vi "Read Current Probe.vi"(0 "object in":refnum<class "TBS2000Series.lvclass">, 2 "Main Channel":i32(ring)=2 items=["Math", "Channel 1", "Channel 2", "Channel 3", "Channel 4"], 3 "Probe Channel":i32(ring)=3 items=["Math", "Channel 1", "Channel 2", "Channel 3", "Channel 4"], 5 "error in (no error)":errorcluster) -> (14 "object out":refnum<class "TBS2000Series.lvclass">, 15 "Phase Probe":dbl format="%.2p", 16 "Peak-to-Peak Probe":dbl format="%.2p", 19 "error out":errorcluster)   [LabVIEW 2023, in "TBS2000Series.lvclass"]
uses:
  TBS2000Series.lvclass
  TBS2000Series.lvclass/TBS2000Series.ctl
  <instrlib>/Tektronix TBS 2000 Series/Tektronix TBS 2000 Series.lvlib
panel:
  out "Waveform Graph":T1(graph)
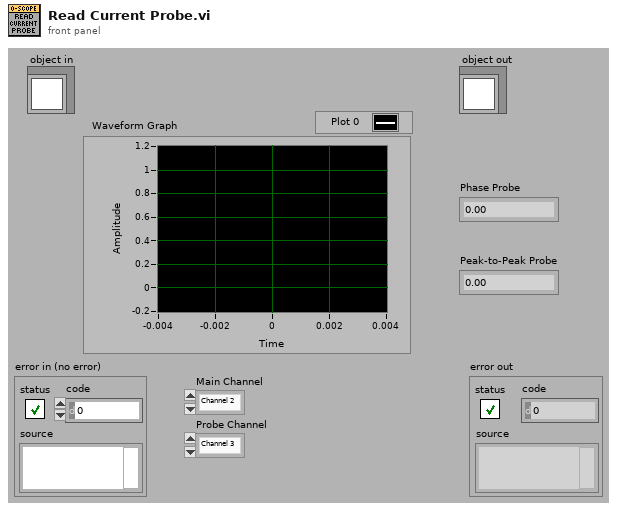
[diagram p1: front panel]
types:
  T1 = cluster{"Initial X":dbl, "X Increment":dbl, "Waveform Array":dbl[]}
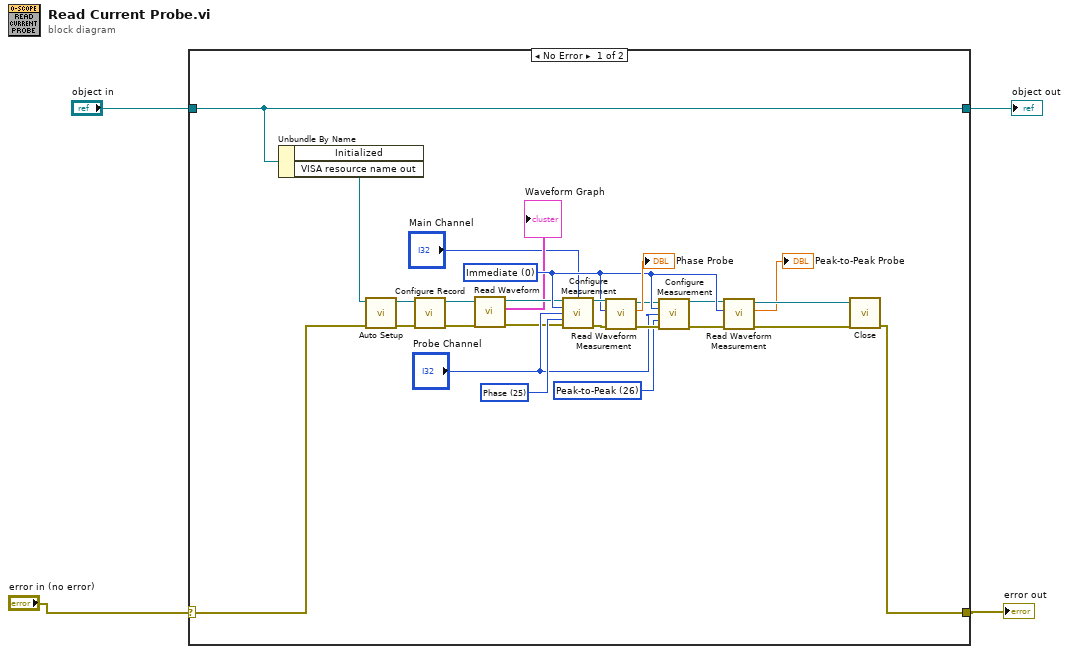
[diagram p0: block diagram]
diagram:
  n1 = case shown="No Error" "error in (no error)" {
    selector: "error in (no error)" -> [w22 w32]
    tunnel: [w21 w32] -> w2
    tunnel: [w23 w31] -> w1
    tunnel: "object in" -> [w23 w31]
    frame No Error {
      w12 = 26 items=["Amplitude", "Area", "Burst", "Cycle Area", "Cycle Mean", "Cycle RMS", "Delay RR", "Delay RF", "Delay FR", "Delay FF", "Fall Time", "Frequency", "High Reference", "Low Reference", "Max", "Mean", "Min", "- Duty Cycle", "- Edge Count", "- Overshoot", "- Pulse Count", "- Width", "+ Duty Cycle", "+ Edge Count", "Period", "Phase", "Peak-to-Peak", "+ Overshoot", "+ Pulse Count", "+ Width", "Rise", "RMS"] ("Measurement Type (30: Rise)")
      w29 = 25 items=["Amplitude", "Area", "Burst", "Cycle Area", "Cycle Mean", "Cycle RMS", "Delay RR", "Delay RF", "Delay FR", "Delay FF", "Fall Time", "Frequency", "High Reference", "Low Reference", "Max", "Mean", "Min", "- Duty Cycle", "- Edge Count", "- Overshoot", "- Pulse Count", "- Width", "+ Duty Cycle", "+ Edge Count", "Period", "Phase", "Peak-to-Peak", "+ Overshoot", "+ Pulse Count", "+ Width", "Rise", "RMS"] ("Measurement Type (0: Amplitude)")
      w16 = 0 items=["Immediate", "Measurement 1", "Measurement 2", "Measurement 3", "Measurement 4", "Measurement 5", "Measurement 6"] ("Measurement Slot")
      n2 = Unbundle By Name(w23) -> ("VISA resource name out"=w26:refnum<visa-resource-name>)  [unwired: 1 out]
      n3 = call <instrlib>:"Auto Setup.vi"("error in (no error)"=w22, "VISA resource name"=w26) -> ("error out"=w24:errorcluster, "VISA resource name out"=w25:refnum<visa-resource-name>)  [unwired: 8 in]
      n4 = call <instrlib>:"Configure Record.vi"("error in (no error)"=w24, "VISA resource name"=w25) -> ("error out"=w8:errorcluster, "VISA resource name out"=w10:refnum<visa-resource-name>)  [unwired: 8 in]
      n5 = call <instrlib>:"Read Waveform.vi"("error in (no error)"=w8, "VISA resource name"=w10) -> ("error out"=w7:errorcluster, "Waveform Graph"=→"Waveform Graph":T1, "VISA resource name out"=w9:refnum<visa-resource-name>)  [unwired: 7 in]
      n6 = call <instrlib>:"Configure Measurement.vi"("VISA resource name"=w9, "Measurement Source 2 (2: Channel 2)"="Main Channel", "Measurement Slot (0: Immediate)"=w16, "Measurement Source 1 (1: Channel 1)"="Probe Channel", "Measurement Type (30: Rise)"=w29, "error in (no error)"=w7) -> ("VISA resource name out"=w28:refnum<visa-resource-name>, "error out"=w27:errorcluster)  [unwired: 8 in]
      n7 = call <instrlib>:"Read Waveform Measurement.vi"("error in (no error)"=w27, "Measurement Slot (0: Immediate)"=w16, "VISA resource name"=w28) -> ("error out"=w17:errorcluster, "Measurement"=→"Phase Probe":dbl, "VISA resource name out"=w15:refnum<visa-resource-name>)  [unwired: 6 in]
      n8 = call <instrlib>:"Configure Measurement.vi"("VISA resource name"=w15, "Measurement Slot (0: Immediate)"=w16, "Measurement Source 1 (1: Channel 1)"="Probe Channel", "Measurement Type (30: Rise)"=w12, "error in (no error)"=w17) -> ("VISA resource name out"=w14:refnum<visa-resource-name>, "error out"=w18:errorcluster)  [unwired: 9 in]
      n9 = call <instrlib>:"Read Waveform Measurement.vi"("error in (no error)"=w18, "Measurement Slot (0: Immediate)"=w16, "VISA resource name"=w14) -> ("error out"=w19:errorcluster, "Measurement"=→"Peak-to-Peak Probe":dbl, "VISA resource name out"=w20:refnum<visa-resource-name>)  [unwired: 6 in]
      n10 = call <instrlib>:"Close.vi"("error in (no error)"=w19, "VISA resource name"=w20) -> ("error out"=w21:errorcluster)  [unwired: 9 in]
    }
    frame Error {
    }
  }
  "error out" <- w2
  "object out" <- w1
